vi "Handle Browse.vi"(7 "Data in":path, 8 "error in (no error)":errorcluster, 11 "Persistent Path Selector in":refnum<class "MGI Persistent Path Selector.lvclass">) -> (0 "error out":errorcluster, 3 "Persistent Path Selector out":refnum<class "MGI Persistent Path Selector.lvclass">, 5 "Data out":path)   [LabVIEW 2020, in "MGI Persistent Path Selector.lvclass"]
doc: "Display Dialog to allow user to select a file.\n\nAuthored by Shawn Walpole\nsupport@mooregoodideas.com\nwww.mooregoodideas.com\n\nCopyright (c) 2013, Moore Good Ideas, Inc.\n\nAll rights reserved.\n\nRedistribution and use in source and binary forms, with or without modification, are permitted provided that the following conditions are met:\n\n * Redistributions of source code must retain the above copyright notice, this list of conditions and the following disclaimer.\n * Redistributions in binary form must reproduce the above copyright notice, this list of conditions and the following disclaimer in the documentation and/or other materials provided with the distribution.\n * Neither the name of Moore Good Ideas, Inc. nor the names of its contributors may be used to endorse or promote products derived from this software without specific prior written permission.\n\nTHIS SOFTWARE IS PROVIDED BY THE COPYRIGHT HOLDERS AND CONTRIBUTORS \"AS IS\" AND ANY EXPRESS OR IMPLIED WARRANTIES, INCLUDING, BUT NOT LIMITED TO, THE IMPLIED WARRANTIES OF MERCHANTABILITY AND FITNESS FOR A PARTICULAR PURPOSE ARE DISCLAIMED. IN NO EVENT SHALL THE COPYRIGHT OWNER OR CONTRIBUTORS BE LIABLE FOR ANY DIRECT, INDIRECT, INCIDENTAL, SPECIAL, EXEMPLARY, OR CONSEQUENTIAL DAMAGES (INCLUDING, BUT NOT LIMITED TO, PROCUREMENT OF SUBSTITUTE GOODS OR SERVICES; LOSS OF USE, DATA, OR PROFITS; OR BUSINESS INTERRUPTION) HOWEVER CAUSED AND ON ANY THEORY OF LIABILITY, WHETHER IN CONTRACT, STRICT LIABILITY, OR TORT (INCLUDING NEGLIGENCE OR OTHERWISE) ARISING IN ANY WAY OUT OF THE USE OF THIS SOFTWARE, EVEN IF ADVISED OF THE POSSIBILITY OF SUCH DAMAGE."
uses:
  <userlib>/_MGI/User Interface/Path Selector XControl/Class Hierarchy/Persistent Path Selector/MGI Persistent Path Selector.lvclass
  <userlib>/_MGI/User Interface/Path Selector XControl/Class Hierarchy/Persistent Path Selector/MGI Persistent Path Selector.lvclass/MGI Persistent Path Selector.ctl
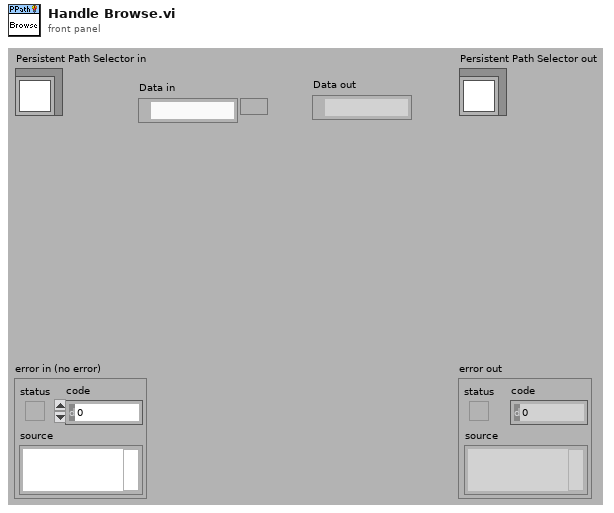
[diagram p1: front panel]
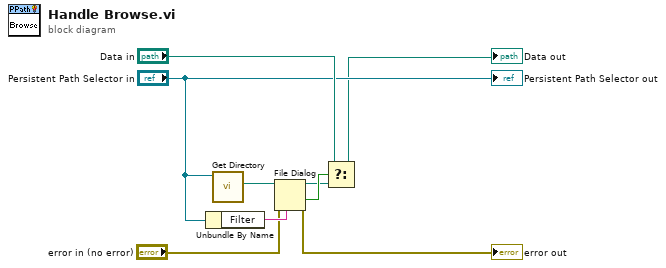
[diagram p0: block diagram]
diagram:
  n1 = Unbundle By Name("Persistent Path Selector in") -> ("Filter"=w6:string)
  n2 = call-dynamic "Get Directory.vi"("Persistent Path Selector"="Persistent Path Selector in") -> ("Start Path"=w9:path)  [unwired: 9 in, 1 out]
  n3 = File Dialog(6:w6, 8:"error in (no error)", 11:w9) -> (0:→"error out":errorcluster, 1:w8:bool, 3:w7:path)  [unwired: 4 in, 1 out]
  n4 = Select(t="Data in", s=w8, f=w7) -> (s? t:f=→"Data out":path)
  "Persistent Path Selector out" <- "Persistent Path Selector in"
